vi "Configure Normalize.vi"(7 "Enable Normalize (T: Enable)":bool=TRUE, 8 "error in (no error)":errorcluster, 9 "Normalized Reference Position (10)":i32=10, 10 "Normalized Reference Level (0 dB)":dbl, 11 "VISA resource name":refnum<visa-resource-name>) -> (0 "error out":errorcluster, 3 "VISA resource name out":refnum<visa-resource-name>)   [LabVIEW 2014, in "Agilent ESA PSA Series.lvlib"]
doc: "Configures normalization functionality."
uses:
  Agilent ESA PSA Series.lvlib
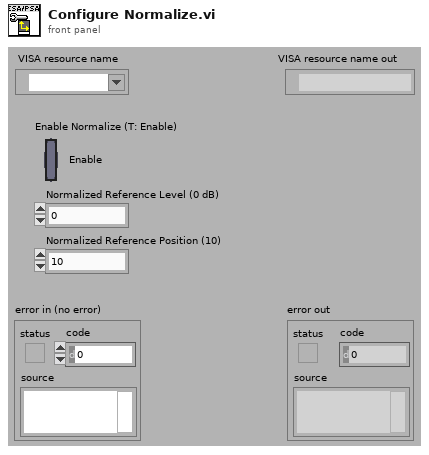
[diagram p1: front panel]
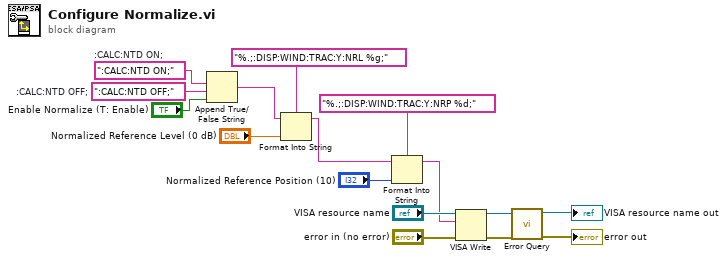
[diagram p0: block diagram]
diagram:
  w8 = ":CALC:NTD ON;"  # :CALC:NTD ON;
  w9 = ":CALC:NTD OFF;"  # :CALC:NTD OFF;
  n1 = Append True/False String(1:"Enable Normalize (T: Enable)", 2:w9, 3:w8) -> (0:w5:string)  [unwired: 1 in]
  n2 = Format Into String(format string="%.;:DISP:WIND:TRAC:Y:NRL %g;", initial string=w5, "Normalized Reference Level (0 dB)") -> (resulting string=w2:string)  [unwired: 1 in, 1 out]
  n3 = Format Into String(format string="%.;:DISP:WIND:TRAC:Y:NRP %d;", initial string=w2, "Normalized Reference Position (10)") -> (resulting string=w1:string)  [unwired: 1 in, 1 out]
  n4 = VISA Write(VISA resource name="VISA resource name", write buffer=w1, error in (no error)="error in (no error)") -> (VISA resource name out=w14:refnum<visa-resource-name>, error out=w12:errorcluster)  [unwired: 1 out]
  n5 = call "Error Query.vi"("error in (no error)"=w12, "VISA resource name"=w14) -> ("error out"=→"error out":errorcluster, "VISA resource name out"=→"VISA resource name out":refnum<visa-resource-name>)  [unwired: 6 in, 2 out]
